vi "ClientSrv Server Module.vi"(5 "LuaVIEW reference":T1, 7 "function index":i32) -> (15 "error out":errorcluster)   [LabVIEW 2012]
doc: "Module required by the \"access.lua\" script. It initializes VI-server security and remote access."
uses:
  luaview/typedefs/t_LuaVIEW Reference.ctl
  typedefs/t_ClientSrv Server Access State Methods.ctl
  luaview/subvis/private/LuaVIEW Pull (string).vi
  luaview/subvis/private/LuaVIEW Pull (refnum).vi
  luaview/subvis/private/LuaVIEW Pull (path).vi
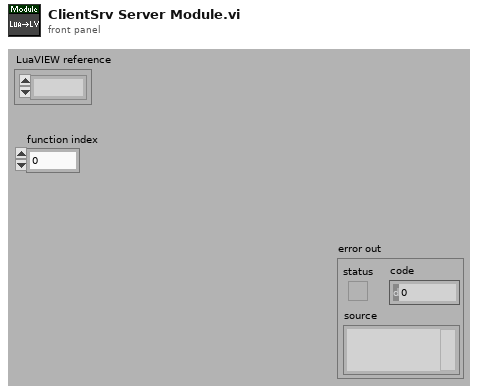
[diagram p1: front panel]
types:
  T1 = typedef "t_LuaVIEW Reference.ctl" = refnum<k1>
  T2 = enum32{"initialize", "open_served_VIs(str:rootpath)", "cleanup()"}
  T3 = typedef "t_ClientSrv Server Access State Methods.ctl" = enum16{"initialize", "validate access", "test access", "release access", "get name", "dummy", "cleanup"}
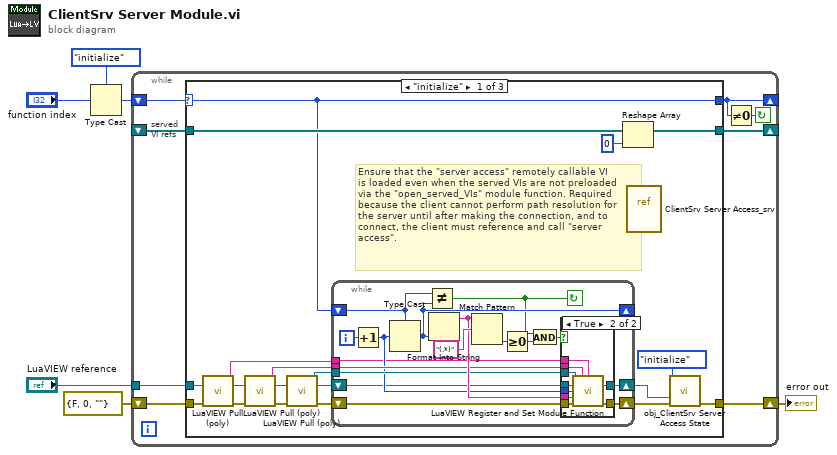
[diagram p0: block diagram]
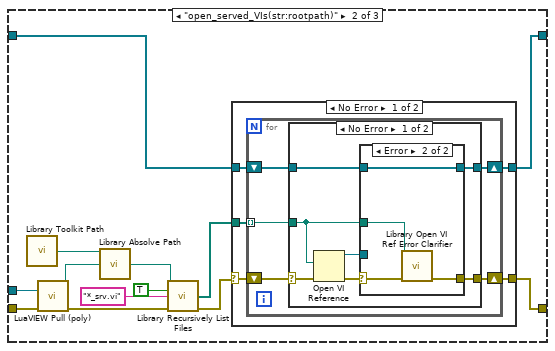
[diagram p3: hidden frame]
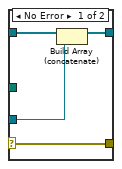
[diagram p4: hidden frame]
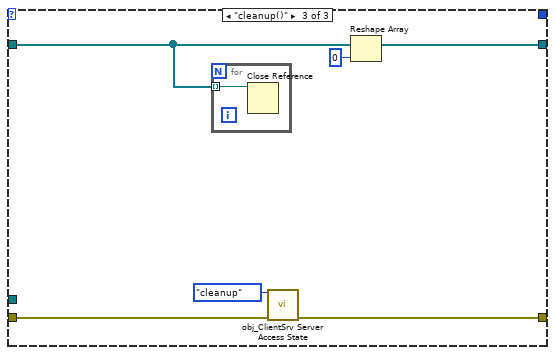
[diagram p7: hidden frame]
diagram:
  n1 = Type Cast(type=T2."initialize" ("cases"), x="function index") -> (*(type *) &x=w5:T2)
  n2 = while {
    shift-right: [w8] -> _
    shift-left: w5 -> [w14]
    shift-right: [w13] -> w6
    shift-left: errorcluster {"status"=FALSE, "code"=0, "source"=""} ("error out") -> [w12]
    shift-right: [w9] -> _
    shift-left: _ -> [w11]
    tunnel: "LuaVIEW reference" -> [w10]
    stop <- w7 continue-if-true
    # "served\nVI refs"
    n3 = case shown="\"initialize\"" w14 {
      selector: w14 -> [w20 _ _]
      tunnel: [w20 _ _] -> w8
      tunnel: w10 -> [w26 w71 _]
      tunnel: [w16 w74 w104] -> w13
      tunnel: w12 -> [w25 w72 w105]
      tunnel: w11 -> [w24 w65 w109]
      tunnel: [w23 w73 w107] -> w9
      frame "initialize" {
        # "Ensure that the \"server access\" remotely callable VI \nis loaded even when the served VIs are not preloaded\nvia the \"open_served_VIs\" module function. Required\nbecause the client cannot perform path resolution for\nthe server until after making the connection, and to\nconnect, the client must reference and call \"server\naccess\"."
        n4 = call-poly "LuaVIEW Pull (poly).vi"("LuaVIEW reference in"=w26, "error in (no error)"=w25) -> ("string"=w29:string, "LuaVIEW reference out"=w31:T1, "error out"=w30:errorcluster)  [unwired: 11 in]
        n5 = call-poly "LuaVIEW Pull (poly).vi"("LuaVIEW reference in"=w31, "error in (no error)"=w30) -> ("string"=w33:string, "LuaVIEW reference out"=w27:T1, "error out"=w28:errorcluster)  [unwired: 11 in]
        n6 = call-poly "LuaVIEW Pull (poly).vi"("LuaVIEW reference in"=w27, "error in (no error)"=w28) -> ("refnum"=w32:refnum<vi>, "LuaVIEW reference out"=w18:T1, "error out"=w19:errorcluster)  [unwired: 11 in]
        n7 = while {
          tunnel: w29 -> [w39]
          shift-right: [w47] -> w17
          shift-left: w19 -> [w48]
          shift-right: [w43] -> _
          shift-left: w20 -> [w44]
          tunnel: w33 -> [w41]
          tunnel: w32 -> [w42]
          shift-right: [w34] -> w15
          shift-left: w18 -> [w35]
          i -> [w46]
          stop <- w36 continue-if-true
          n8 = Increment(x=w46) -> (x+1=w40:i32)
          n9 = Type Cast(type=w44, x=w40) -> (*(type *) &x=w43:T2)
          n10 = Not Equal?(x=w44, y=w43) -> (x != y?=w36:bool)
          n11 = Format Into String(w43) -> (resulting string=w45:string)  [unwired: 3 in, 1 out]
          n12 = Match Pattern(string=w45, regular expression="(.*)") -> (offset past match=w49:i32)  [unwired: 1 in, 3 out]
          n13 = Greater Or Equal To 0?(x=w49) -> (x >= 0?=w38:bool)
          n14 = And(x=w36, y=w38) -> (x .and. y?=w37:bool)
          n15 = case shown="True" w37 {
            tunnel: w39 -> [_ w55]
            tunnel: w35 -> [w51 w59]
            tunnel: w40 -> [_ w60]
            tunnel: w45 -> [_ w57]
            tunnel: [w52 w61] -> w47
            tunnel: w48 -> [w52 w58]
            tunnel: w41 -> [_ w56]
            tunnel: w42 -> [_ w54]
            tunnel: [w51 w53] -> w34
            frame False {
            }
            frame True {
              n16 = call "LuaVIEW Register and Set Module Function.vi"("module refnum"=w54, "export table (set as global)"=w56, "table (set as global)"=w55, "LuaVIEW reference in"=w59, "index"=w60, "synopsis"=w57, "error in (no error)"=w58) -> ("LuaVIEW reference out"=w53:T1, "error out"=w61:errorcluster)  [unwired: 7 in]
            }
          }
        }
        n17 = Reshape Array(w24, 0 ("dimension size")) -> (w23:refnum<vi>[])
        n18 = vi-ref "ClientSrv Server Access_srv.vi"() -> ()  [unwired: 1 out]
        n19 = call "obj_ClientSrv Server Access State.vi"("method (test access)"=t_ClientSrv_Server_Access_State_Methods."initialize", "LuaVIEW reference {initialize}"=w15, "error in (no error)"=w17) -> ("error out"=w16:errorcluster)  [unwired: 10 in, 2 out]
      }
      frame "open_served_VIs(str:rootpath)" {
        n20 = call "Library Toolkit Path.vi"() -> ("absolute toolkit path"=w64:path)  [unwired: 15 in]
        n21 = call-poly "LuaVIEW Pull (poly).vi"("LuaVIEW reference in"=w71, "error in (no error)"=w72) -> ("path"=w63:path, "error out"=w68:errorcluster)  [unwired: 11 in, 1 out]
        n22 = call "Library Absolve Path.vi"("absolute base"=w64, "input path to absolve"=w63) -> ("absolved path"=w62:path)  [unwired: 13 in]
        n23 = call "Library Recursively List Files.vi"("root directory"=w62, "enter llbs? (no)"=TRUE, "pattern (none)"="*_srv.vi", "error in (no error)"=w68) -> ("file list"=w66:path[], "error out"=w67:errorcluster)  [unwired: 9 in, 1 out]
        n24 = case shown="No Error" w67 {
          selector: w67 -> [w79 w103]
          tunnel: [w77 w103] -> w74
          tunnel: w66 -> [w78 _]
          tunnel: w65 -> [w76 w102]
          tunnel: [w75 w102] -> w73
          frame No Error {
            n25 = for {
              shift-right: [w82] -> w77
              shift-left: w79 -> [w83]
              tunnel: w78 -> [w84] mode=indexing
              shift-right: [w81] -> w75
              shift-left: w76 -> [w80]
              n26 = case shown="No Error" w83 {
                selector: w83 -> [w90 w101]
                tunnel: w84 -> [w86 _]
                tunnel: [w85 w101] -> w82
                tunnel: [w88 w100] -> w81
                tunnel: w80 -> [w87 w100]
                frame No Error {
                  n27 = Open VI Reference(vi path=w86, error in (no error)=w90) -> (vi reference=w89:refnum<vi>, error out=w91:errorcluster)  [unwired: 4 in]
                  n28 = case shown="Error" w91 {
                    selector: w91 -> [w92 w98]
                    tunnel: w89 -> [w95 _]
                    tunnel: [w94 w99] -> w88
                    tunnel: w87 -> [w93 w99]
                    tunnel: w86 -> [_ w96]
                    tunnel: [w92 w97] -> w85
                    frame No Error {
                      n29 = Build Array (concatenate)(w93, w95) -> (w94:refnum<vi>[])
                    }
                    frame Error {
                      n30 = call "Library Open VI Ref Error Clarifier.vi"("VI path"=w96, "called VI error (no error)"=w98) -> ("error out"=w97:errorcluster)  [unwired: 13 in]
                    }
                  }
                }
                frame Error {
                }
              }
            }
          }
          frame Error {
          }
        }
      }
      frame "cleanup()" {
        n31 = for {
          tunnel: w109 -> [w110] mode=indexing
          n32 = Close Reference(reference=w110) -> ()  [unwired: 1 in, 1 out]
        }
        n33 = call "obj_ClientSrv Server Access State.vi"("method (test access)"=t_ClientSrv_Server_Access_State_Methods."cleanup" ("method"), "error in (no error)"=w105) -> ("error out"=w104:errorcluster)  [unwired: 11 in, 2 out]
        n34 = Reshape Array(w109, 0 ("dimension size")) -> (w107:refnum<vi>[])
      }
    }
    n35 = Not Equal To 0?(x=w8) -> (x != 0?=w7:bool)
  }
  "error out" <- w6
